vi "myRIO v1.0 Reserve Channel List.vi"(7 "Allow multiple opens?":bool, 8 "error in (no error)":errorcluster, 10 "Channel Reservation List":T1, 11 "Owner":string) -> (0 "error out":errorcluster)   [LabVIEW 2021]
uses:
  <vilib>/myRIO/Common/Instrument Driver Framework/myRIO v1.0/Resource Manager/typedefs/myRIO v1.0 Channel Reservation List.ctl
  <vilib>/myRIO/Common/Instrument Driver Framework/myRIO v1.0/Resource Manager/typedefs/myRIO v1.0 Channel Reservation Info.ctl
  <vilib>/myRIO/Common/Instrument Driver Framework/myRIO v1.0/Resource Manager/typedefs/myRIO v1.0 Connector List.ctl
  <vilib>/myRIO/Common/Instrument Driver Framework/myRIO v1.0/Resource Manager/vis/myRIO v1.0 Build Mutex Name.vi
  <vilib>/myRIO/Common/Instrument Driver Framework/Utilities/vis/IO Manager.vi
  <vilib>/Utility/error.llb/Error Cluster From Error Code.vi
  <vilib>/myRIO/Common/Instrument Driver Framework/Utilities/vis/Configuration Manager.vi
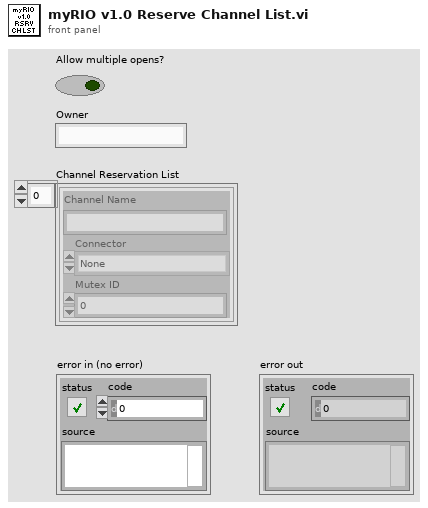
[diagram p1: front panel]
types:
  T1 = typedef "myRIO v1.0 Channel Reservation List.ctl" = T2[]
  T2 = typedef "myRIO v1.0 Channel Reservation Info.ctl" = cluster{"Channel Name":string, "Connector":T3, "Mutex ID":i32}
  T3 = typedef "myRIO v1.0 Connector List.ctl" = enum32{"None", "ConnectorA", "ConnectorB", "ConnectorC"}
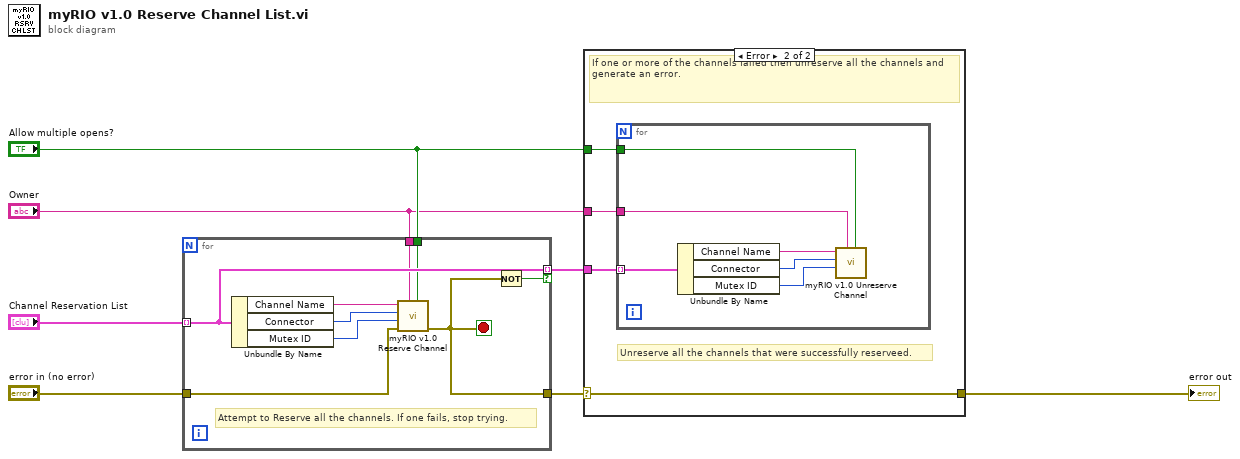
[diagram p0: block diagram]
diagram:
  n1 = for {
    tunnel: "Allow multiple opens?" -> [w14]
    tunnel: [w9] -> w7
    tunnel: "Channel Reservation List" -> [w16] mode=indexing
    tunnel: [w16] -> w5 mode=indexing if=w15
    tunnel: "Owner" -> [w13]
    tunnel: "error in (no error)" -> [w8]
    stop <- w9 stop-if-true
    # "Attempt to Reserve all the channels. If one fails, stop trying."
    n2 = Unbundle By Name(w16) -> ("Channel Name"=w12:string, "Connector"=w11:T3, "Mutex ID"=w10:i32)
    n3 = call <vilib>:"myRIO v1.0 Reserve Channel.vi"("Allow multiple opens?"=w14, "Owner"=w13, "error in (no error)"=w8, "Mutex ID"=w10, "Connector"=w11, "Channel Name"=w12) -> ("error out"=w9:errorcluster)  [unwired: 5 in]
    n4 = Not(x=w9) -> (.not. x?=w15:bool)
  }
  n5 = case shown="Error" w7 {
    selector: w7 -> [w17 w18]
    tunnel: w5 -> [_ w21]
    tunnel: "Owner" -> [_ w20]
    tunnel: "Allow multiple opens?" -> [_ w19]
    tunnel: [w17 w18] -> w3
    frame No Error {
      # "If all channels were successfully reserved then there is nothing to do."
    }
    frame Error {
      # "Unreserve all the channels that were successfully reserveed."
      # "If one or more of the channels failed then unreserve all the channels and generate an error."
      n6 = for {
        tunnel: w21 -> [w27] mode=indexing
        tunnel: w20 -> [w25]
        tunnel: w19 -> [w26]
        n7 = Unbundle By Name(w27) -> ("Channel Name"=w24:string, "Connector"=w23:T3, "Mutex ID"=w22:i32)
        n8 = call <vilib>:"myRIO v1.0 Unreserve Channel.vi"("Allow multiple opens?"=w26, "Owner"=w25, "Mutex ID"=w22, "Connector"=w23, "Channel Name"=w24) -> ()  [unwired: 6 in, 1 out]
      }
    }
  }
  "error out" <- w3
